vi "Update Loaded Plugins.vi"(8 "error in (no error)":errorcluster, 11 "CIF_UI in":refnum<class "CIF_Manager_UI.lvclass">) -> (0 "error out":errorcluster)   [LabVIEW 2021, in "CIF_Manager_UI.lvclass"]
uses:
  CIF_Manager_UI.lvclass
  C:/Program Files/National Instruments/LabVIEW 2021/vi.lib/CIF Foundation/CIF Core/CIFUI/CIF_UI.lvclass
  CIF_Manager_UI.lvclass/CIF_Manager_UI.ctl
  <vilib>/CIF Foundation/CIF Core/CIFUI/CIF_UI.lvclass/CIF_UI.ctl
  <vilib>/CIF Foundation/CIF Core/CIFUI/Utilities/Get Plugin Summary Info.vi/3cb97bbe-ec67-4187-806b-96be001ee38f.vi
  <vilib>/Comparison/Less/Less Functor/Less Functor.lvclass
  <vilib>/CIF Foundation/CIF Core/CIFUI/CIF_UI.lvclass
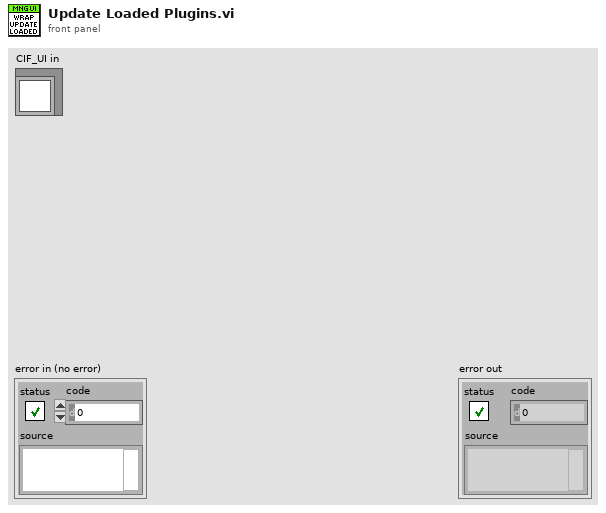
[diagram p1: front panel]
types:
  T1 = typedef "CIF_UI.lvclass/Plugin Summary.ctl" = cluster{"Name":string, "Type":string, "grpc_port":i32, "Version":T2}
  T2 = typedef "CIFCoreCommon.lvlib/Version Simple.ctl" = cluster{"Major":i32, "Minor":i32, "Fix":i32}
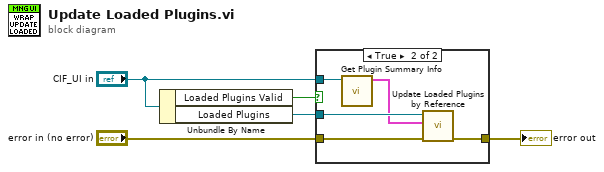
[diagram p0: block diagram]
diagram:
  n1 = Unbundle By Name("CIF_UI in") -> ("Loaded Plugins Valid"=w5:bool, "Loaded Plugins"=w4:refnum<vi>)
  n2 = case shown="True" w5 {
    tunnel: w4 -> [_ w11]
    tunnel: "error in (no error)" -> [w6 w10]
    tunnel: [w6 w9] -> w3
    tunnel: "CIF_UI in" -> [_ w8]
    frame False {
    }
    frame True {
      n3 = call <vilib>:"Get Plugin Summary Info.vi"("CIF_UI in"=w8) -> ("Plugin Summary Info"=w7:T1[])  [unwired: 10 in]
      n4 = call "Update Loaded Plugins by Reference.vi"("error in (no error)"=w10, "Plugin Summary Info"=w7, "Loaded Plugins ref in"=w11) -> ("error out"=w9:errorcluster)  [unwired: 7 in, 1 out]
    }
  }
  "error out" <- w3
